vi "Window Function Generator.vi"(10 "Enum":enum16{"None", "Hanning", "Hamming"}(ring)=enum."Hamming") -> (2 "Window Array":fxp<+,8,1>[](array[numeric]))   [LabVIEW 2014]
uses:
  <vilib>/Analysis/4window.llb/Hanning Window (DBL).vi
  <vilib>/Analysis/4window.llb/Hamming Window (DBL).vi
  <vilib>/Analysis/4window.llb/AllCosWindow (DBL).vi
  <vilib>/Analysis/NI_AALPro.lvlib
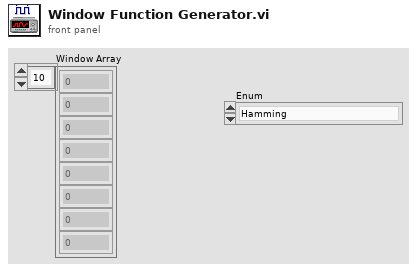
[diagram p1: front panel]
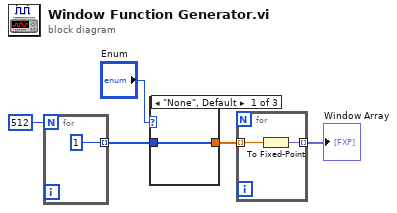
[diagram p0: block diagram]
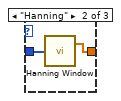
[diagram p2: hidden frame]
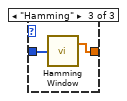
[diagram p3: hidden frame]
diagram:
  n1 = for {
    N: 512 -> [_]
    tunnel: [1] -> w5 mode=indexing
  }
  n2 = case shown="\"None\", Default" "Enum" {
    tunnel: w5 -> [w7 w9 w10]
    tunnel: [w7 w8 w11] -> w2
    frame "None", Default {
    }
    frame "Hanning" {
      n3 = call-poly <vilib>:"Hanning Window.vi"("X"=w9) -> ("Windowed X"=w8:dbl[])  [unwired: 1 out]
    }
    frame "Hamming" {
      n4 = call-poly <vilib>:"Hamming Window.vi"("X"=w10) -> ("Windowed X"=w11:dbl[])  [unwired: 1 out]
    }
  }
  n5 = for {
    tunnel: w2 -> [w13] mode=indexing
    tunnel: [w12] -> w3 mode=indexing
    n6 = To Fixed-Point(number=w13) -> (fixed-point=w12:fxp<+,8,1>)  [unwired: 1 in]
  }
  "Window Array" <- w3
